vi "Configure.vi"(8 "error in (no error)":errorcluster, 10 "Network Stream Writer IP":string, 11 "DataReceiver in":refnum<class "DataReceiver.lvclass">) -> (0 "error out":errorcluster, 3 "DataReceiver out":refnum<class "DataReceiver.lvclass">)   [LabVIEW 2010, in "DataReceiver.lvclass"]
uses:
  DataReceiver.lvclass
  DataReceiver.lvclass/DataReceiver.ctl
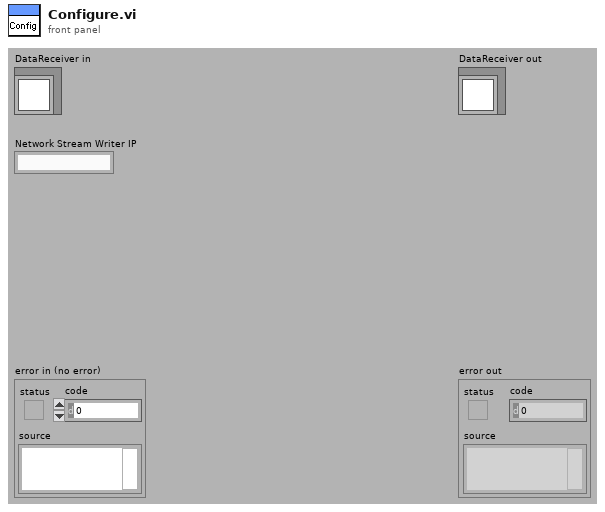
[diagram p1: front panel]
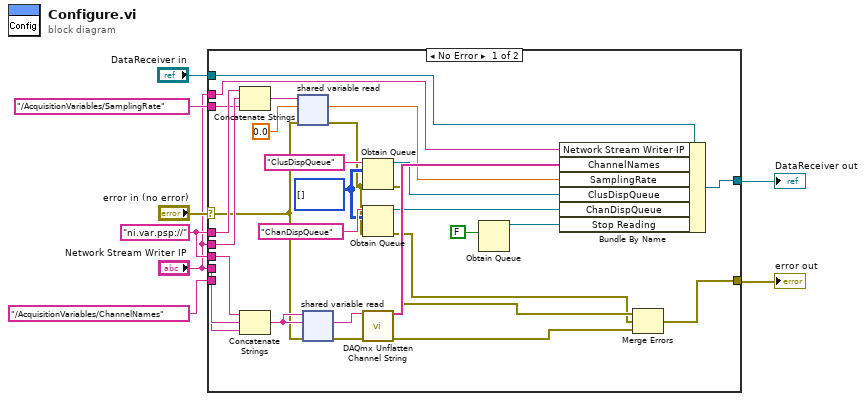
[diagram p0: block diagram]
diagram:
  w3 = "ni.var.psp://" ("string")
  n1 = case shown="No Error" "error in (no error)" {
    selector: "error in (no error)" -> [w28 w39]
    tunnel: [w11 w39] -> w7
    tunnel: [w17 w38] -> w5
    tunnel: "DataReceiver in" -> [w27 w38]
    tunnel: "Network Stream Writer IP" -> [w37 _]
    tunnel: w3 -> [w34 _]
    tunnel: "/AcquisitionVariables/ChannelNames" ("string") -> [w33 _]
    tunnel: "Network Stream Writer IP" -> [w32 _]
    tunnel: w3 -> [w31 _]
    tunnel: "/AcquisitionVariables/SamplingRate" ("string") -> [w30 _]
    tunnel: "Network Stream Writer IP" -> [w16 _]
    frame No Error {
      w20 = i32[][] []
      n2 = Concatenate Strings(w31, w32, w30) -> (w35:string)
      n3 = Concatenate Strings(w34, w37, w33) -> (w36:string)
      n4 = shared-variable-read(w35, w28, 0.0) -> (w15:errorcluster, w23:dbl)  [unwired: 2 out]
      n5 = shared-variable-read(w36, w28, w36) -> (w25:errorcluster, w26:string)  [unwired: 2 out]
      n6 = Obtain Queue(name (unnamed)="ClusDispQueue", element data type=w20, error in (no error)=w15) -> (queue out=w19:refnum<queue>, error out=w14:errorcluster)  [unwired: 2 in, 1 out]
      n7 = Obtain Queue(name (unnamed)="ChanDispQueue", element data type=w20, error in (no error)=w15) -> (queue out=w18:refnum<queue>, error out=w13:errorcluster)  [unwired: 2 in, 1 out]
      n8 = call <vilib>:"DAQmx Unflatten Channel String.vi"("names in"=w26, "error in"=w25) -> ("names out"=w24:string[], "error out"=w12:errorcluster)  [unwired: 12 in]
      n9 = Obtain Queue(element data type=FALSE) -> (queue out=w9:refnum<queue>)  [unwired: 4 in, 2 out]
      n10 = Bundle By Name(cluster=w27, "Network Stream Writer IP"=w16, "ChannelNames"=w24, "SamplingRate"=w23, "ClusDispQueue"=w19, "ChanDispQueue"=w18, "Stop Reading"=w9) -> (w17:refnum<class "DataReceiver.lvclass">)
      n11 = Merge Errors(w14, w13, w12) -> (w11:errorcluster)
    }
    frame Error {
    }
  }
  "error out" <- w7
  "DataReceiver out" <- w5
